vi "MazeGen Path.vi"() -> (3 "MazeGen Path":path)   [LabVIEW 2020, in "App.lvlib" / "MazeUI.lvclass"]
uses:
  MazeUI.lvclass
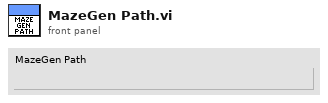
[diagram p1: front panel]
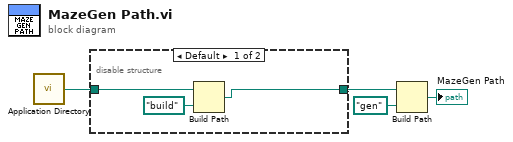
[diagram p0: block diagram]
diagram:
  n1 = call <vilib>:"Application Directory.vi"() -> ("Application Directory"=w4:path)
  n2 = disable-structure shown="Default" {
    disable-tunnel: w4 -> [w7 w8]
    disable-tunnel: [w5 w8] -> w3
    frame condition #0 (active) {
      n3 = Build Path(base path=w7, name or relative path=path "build") -> (appended path=w5:path)
    }
    frame condition #1 {
    }
  }
  n4 = Build Path(base path=w3, name or relative path=path "gen") -> (appended path=→"MazeGen Path":path)
